vi "Module Init.vi"(8 "error in (no error)":errorcluster, 11 "Data Logger Module in":refnum<class "Data Logger Module.lvclass">) -> (0 "error out":errorcluster, 3 "Data Logger Module out":refnum<class "Data Logger Module.lvclass">)   [LabVIEW 2020, in "VolatusData.lvlib" / "Data Logger Module.lvclass"]
uses:
  Data Logger Module.lvclass
  C:/dev/lv20CE/relink/lv-volatus/Volatus/Module/Module.lvclass
  Volatus/Module/Module.lvclass/Module.ctl
  Register Logger.ctl
  Volatus/MessageQ/MessageQ.lvclass
  Data Logger Module.lvclass/Data Logger Module.ctl
  Volatus/MessageQ/MessageQ.lvclass/MessageQ.ctl
  Log Manager Identity/Log Manager Identity.lvclass
  C:/dev/lv20CE/relink/lv-volatus/Volatus/Identity/Identity.lvclass
  Volatus/VolatusAPI/VolatusAPI.lvclass
  Volatus/Module/Module.lvclass
  VolatusData.lvlib
  C:/dev/lv20CE/relink/lv-volatus/VolatusData/Data Logger Module/Data Logger Module.lvclass
  C:/dev/lv20CE/relink/lv-volatus/VolatusData/Log Manager Identity/Log Manager Identity.lvclass
  Logger State.ctl
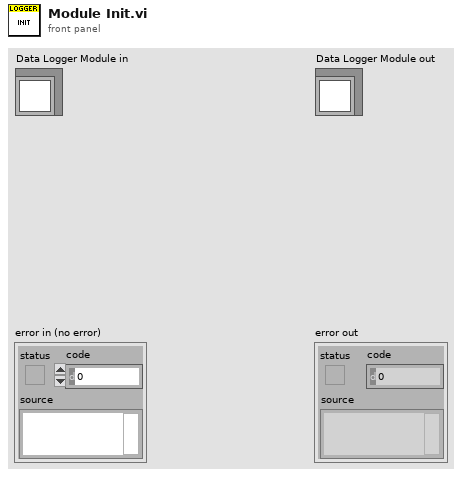
[diagram p1: front panel]
types:
  T1 = typedef "VolatusData.lvlib/Logger State.ctl" = enum16{"Unknown", "Idle", "Preparing", "Ready", "Logging", "Stopping"}
  T2 = typedef "VolatusData.lvlib/Register Logger.ctl" = cluster{"MsgQ":refnum<class "MessageQ.lvclass">, "ID":string, "Group":string}
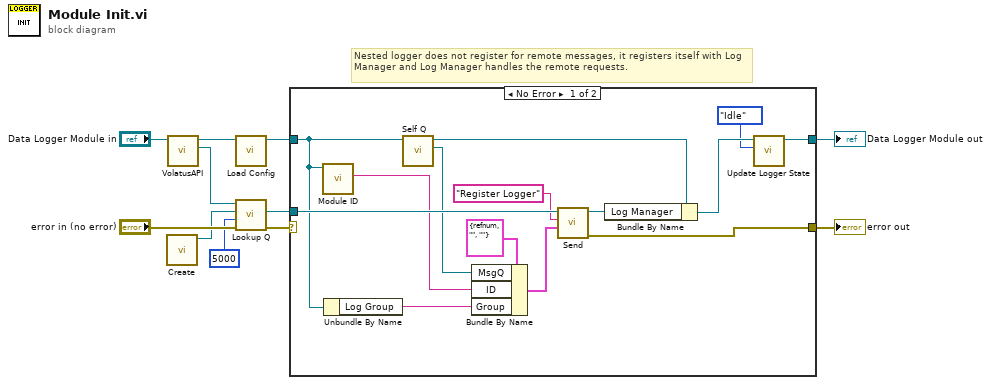
[diagram p0: block diagram]
diagram:
  # "Nested logger does not register for remote messages, it registers itself with Log Manager and Log Manager handles the remote requests."
  n1 = call "Create.vi"() -> ("Log Manager Identity out"=w7:refnum<class "Log Manager Identity.lvclass">)  [unwired: 11 in]
  n2 = call "VolatusAPI.vi"("Module in"="Data Logger Module in") -> ("VolatusAPI"=w8:refnum<class "VolatusAPI.lvclass">, "Module out"=w4:refnum<class "Data Logger Module.lvclass">)  [unwired: 9 in]
  n3 = call "Load Config.vi"("Data Logger Module in"=w4) -> ("Data Logger Module out"=w1:refnum<class "Data Logger Module.lvclass">)  [unwired: 9 in, 1 out]
  n4 = call "Lookup Q.vi"("error in (no error)"="error in (no error)", "Timeout ms (0)"=5000, "Identity"=w7, "VolatusAPI in"=w8) -> ("error out"=w6:errorcluster, "MessageQ"=w5:refnum<class "MessageQ.lvclass">)  [unwired: 5 in, 1 out]
  n5 = case shown="No Error" w6 {
    selector: w6 -> [_ w27]
    tunnel: w5 -> [w25 _]
    tunnel: w1 -> [w15 w26]
    tunnel: [w13 w26] -> w3
    tunnel: [w18 w27] -> w2
    frame No Error {
      n6 = call-dynamic "Module ID.vi"("Data Logger Module in"=w15) -> ("Module ID"=w20:string)  [unwired: 10 in]
      n7 = Unbundle By Name(w15) -> ("Log Group"=w14:string)
      n8 = call "Self Q.vi"("Module in"=w15) -> ("Self Q"=w21:refnum<class "MessageQ.lvclass">, "Module out"=w19:refnum<class "Data Logger Module.lvclass">)  [unwired: 9 in]
      n9 = Bundle By Name(cluster=T2 {"MsgQ"=refnum, "ID"="", "Group"=""} ("Logger Registration"), "MsgQ"=w21, "ID"=w20, "Group"=w14) -> (w22:T2)
      n10 = call "Send.vi"("Data"=w22, "ID"="Register Logger", "MessageQ in"=w25) -> ("error out"=w18:errorcluster, "MessageQ out"=w16:refnum<class "MessageQ.lvclass">)  [unwired: 7 in]
      n11 = Bundle By Name(cluster=w19, "Log Manager"=w16) -> (w17:refnum<class "Data Logger Module.lvclass">)
      n12 = call "Update Logger State.vi"("Logger State"=Logger_State."Idle", "Module in"=w17) -> ("Module"=w13:refnum<class "Data Logger Module.lvclass">)  [unwired: 8 in, 1 out]
    }
    frame Error {
    }
  }
  "error out" <- w2
  "Data Logger Module out" <- w3
